vi "PH_PP_CurrentMeas.set i Attr.vi"(0 "i ref in":refnum<vi>, 5 "error in (no error)":errorcluster) -> (14 "i ref out":refnum<vi>, 17 "i Attributes":T1={"Status"={"GUI Ref Hardware Feedback"=refnum, "Tab Control"=refnum}, "PU 1"={"Instance"="N/A", "Status"=0, "Ref Status "=refnum, "Data"=[], "Ref Data"=refnum}, "PU 2"={"Instance"="N/A", "Status"=0, "Ref Status "=refnum, "Data"=[], "Ref Data"=refnum}, "PU 3"={"Instance"="N/A", "Status"=0, "Ref Status "=refnum, "Data"=[], "Ref Data"=refnum}, "PU 4"={"Instance"="N/A", "Status"=0, "Ref Status "=refnum, "Data"=[], "Ref Data"=refnum}, "PU 5"={"Instance"="N/A", "Status"=0, "Ref Status "=refnum, "Data"=[], "Ref Data"=refnum}, "FR"={"Instance"="N/A", "Status"=0, "Ref Status "=refnum, "Data"=[], "Ref Data"=refnum}, "PA - 19mm 1"={"Instance"="N/A", "Status"=0, "Ref Status "=refnum}, "PA - 19mm 2"={"Instance"="N/A", "Status"=0, "Ref Status "=refnum, "no link"=FALSE}, "PA - 45mm"={"Instance"="N/A", "Status"=0, "Ref Status "=refnum, "no link"=FALSE}, "PA Data"={"Data"=[], "Ref"=refnum}, "Sequencer"={"Instance"="N/A", "SM State Ref"=refnum}, "Tasks"=[], "in use"={"MA DP"=FALSE, "FR and PA"=FALSE}, "DAQ Server"="N/A"} {"Tasks"."Status" items=["no info", "off/false/out", "on/true/in", "Failure", "Alarm", "Status 1", "Status 2", "Status 3"]; "PA - 45mm"."Status" items=["no info", "off/false/out", "on/true/in", "Failure", "Alarm", "Status 1", "Status 2", "Status 3"]; "PA - 19mm 2"."Status" items=["no info", "off/false/out", "on/true/in", "Failure", "Alarm", "Status 1", "Status 2", "Status 3"]; "PA - 19mm 1"."Status" items=["no info", "off/false/out", "on/true/in", "Failure", "Alarm", "Status 1", "Status 2", "Status 3"]; "FR"."Status" items=["no info", "off/false/out", "on/true/in", "Failure", "Alarm", "Status 1", "Status 2", "Status 3"]; "PU 5"."Status" items=["no info", "off/false/out", "on/true/in", "Failure", "Alarm", "Status 1", "Status 2", "Status 3"]; "PU 4"."Status" items=["no info", "off/false/out", "on/true/in", "Failure", "Alarm", "Status 1", "Status 2", "Status 3"]; "PU 3"."Status" items=["no info", "off/false/out", "on/true/in", "Failure", "Alarm", "Status 1", "Status 2", "Status 3"]; "PU 2"."Status" items=["no info", "off/false/out", "on/true/in", "Failure", "Alarm", "Status 1", "Status 2", "Status 3"]; "PU 1"."Status" items=["no info", "off/false/out", "on/true/in", "Failure", "Alarm", "Status 1", "Status 2", "Status 3"]}, 19 "error out":errorcluster)   [LabVIEW 2014, in "PH_PP_CurrentMeas.lvlib"]
doc: "Within this VI several Attributes are set the first time."
uses:
  PH_PP_CurrentMeas.lvlib
  PH_PP_CurrentMeas.i attribute.ctl
  PH_Basics/PH_StatusHandler/PH_StatusHandler.Status.ctl
  PH_Basics/PH_StatusHandler/PH_StatusHandler.GUI element.ctl
  PH_PP_CurrentMeas.CommandCluster.ctl
  PH_Basics/PH_StatusHandler/PH_StatusHandler.lvlib
  PH_Basics/PH_Common/PH_Common.lvlib
  CS_Core/CSSystem/CSSystemLib/CSSystemLib.lvlib
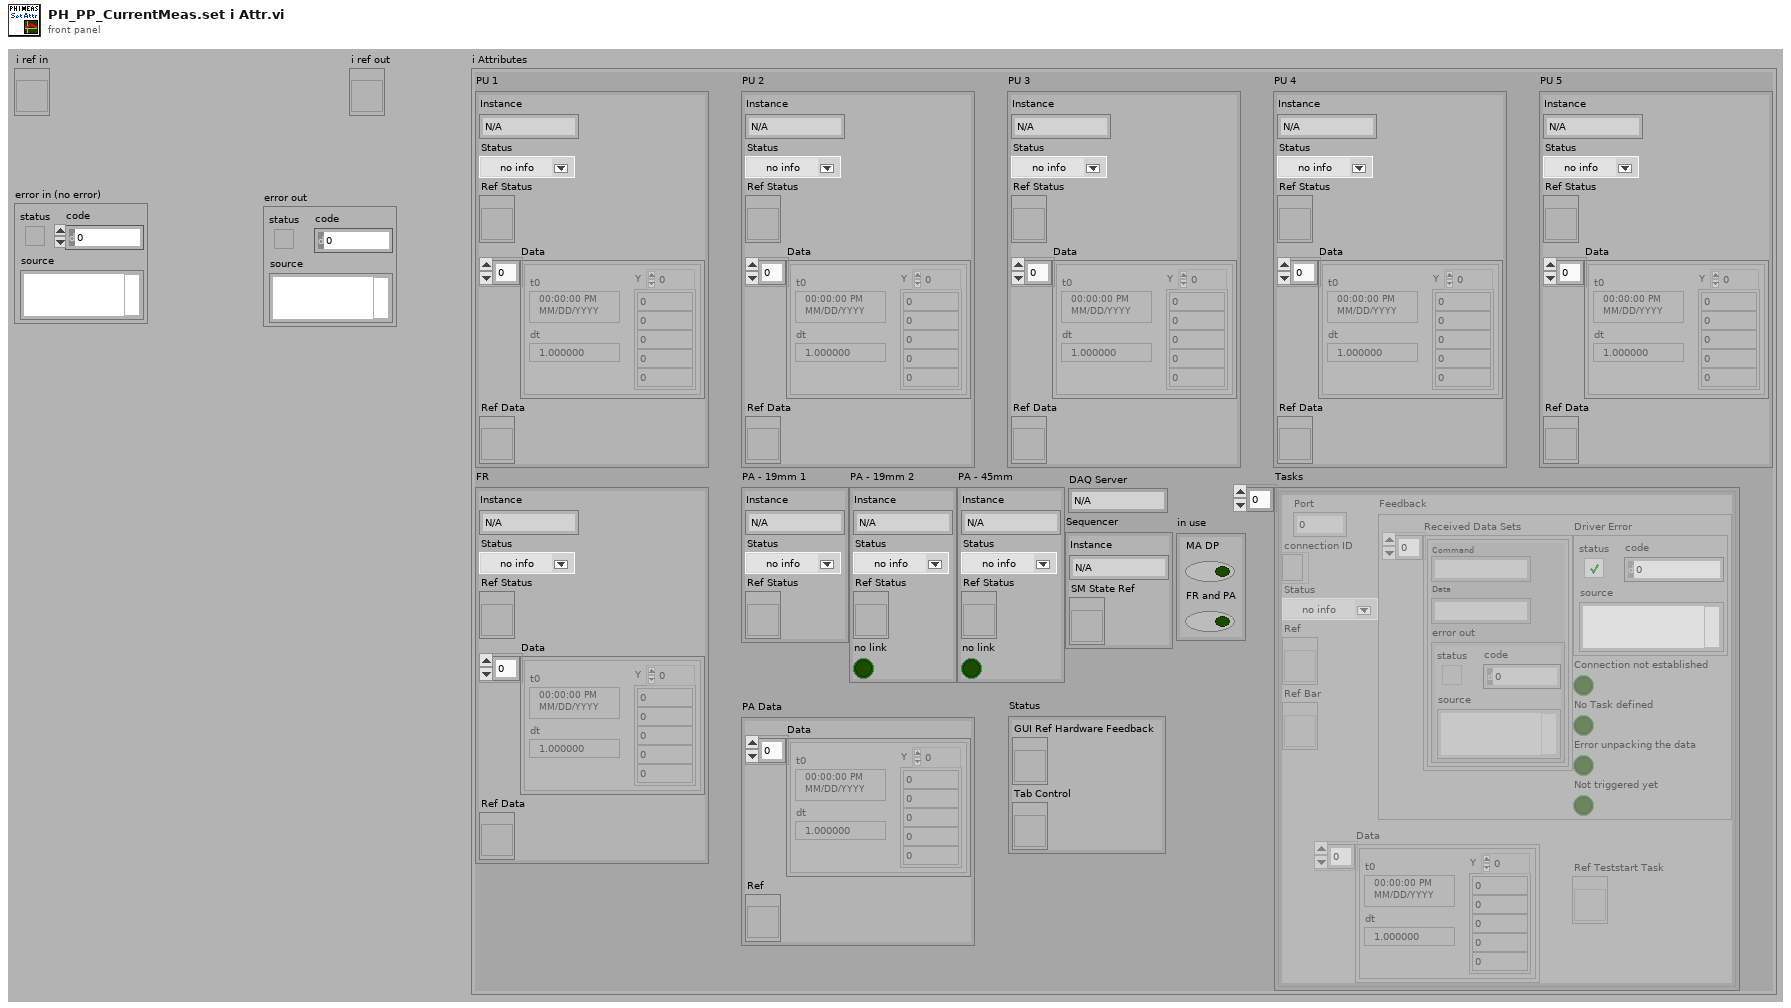
[diagram p1: front panel]
types:
  T1 = typedef "PH_PP_CurrentMeas.lvlib/PH_PP_CurrentMeas.i attribute.ctl" = cluster{"Status":cluster{"GUI Ref Hardware Feedback":refnum<vi>, "Tab Control":refnum<vi>}, "PU 1":cluster{"Instance":string, "Status":T2, "Ref Status ":refnum<vi>, "Data":waveform(dbl)[], "Ref Data":refnum<vi>}, "PU 2":cluster{"Instance":string, "Status":T2, "Ref Status ":refnum<vi>, "Data":waveform(dbl)[], "Ref Data":refnum<vi>}, "PU 3":cluster{"Instance":string, "Status":T2, "Ref Status ":refnum<vi>, "Data":waveform(dbl)[], "Ref Data":refnum<vi>}, "PU 4":cluster{"Instance":string, "Status":T2, "Ref Status ":refnum<vi>, "Data":waveform(dbl)[], "Ref Data":refnum<vi>}, "PU 5":cluster{"Instance":string, "Status":T2, "Ref Status ":refnum<vi>, "Data":waveform(dbl)[], "Ref Data":refnum<vi>}, "FR":cluster{"Instance":string, "Status":T2, "Ref Status ":refnum<vi>, "Data":waveform(dbl)[], "Ref Data":refnum<vi>}, "PA - 19mm 1":cluster{"Instance":string, "Status":T2, "Ref Status ":refnum<vi>}, "PA - 19mm 2":cluster{"Instance":string, "Status":T2, "Ref Status ":refnum<vi>, "no link":bool}, "PA - 45mm":cluster{"Instance":string, "Status":T2, "Ref Status ":refnum<vi>, "no link":bool}, "PA Data":cluster{"Data":waveform(dbl)[], "Ref":refnum<vi>}, "Sequencer":cluster{"Instance":string, "SM State Ref":refnum<vi>}, "Tasks":cluster{"Port":u16, "connection ID":refnum<k5>, "Status":T2, "Ref":refnum<vi>, "Ref Bar":refnum<vi>, "Feedback":cluster{"Received Data Sets":T3[], "Driver Error":errorcluster, "Connection not established":bool, "Error unpacking the data":bool, "No Task defined":bool, "Not triggered yet":bool}, "Data":waveform(dbl)[], "Ref Teststart Task":refnum<vi>}[], "in use":cluster{"MA DP":bool, "FR and PA":bool}, "DAQ Server":string}
  T2 = typedef "PH_StatusHandler.lvlib/PH_StatusHandler.Status.ctl" = i16
  T3 = typedef "PH_PP_CurrentMeas.lvlib/PH_PP_CurrentMeas.CommandCluster.ctl" = cluster{"Command":string, "Data":string, "error out":errorcluster}
  T4 = cluster{"Port":u16, "connection ID":refnum<k5>, "Status":T2, "Ref":refnum<vi>, "Ref Bar":refnum<vi>, "Feedback":cluster{"Received Data Sets":T3[], "Driver Error":errorcluster, "Connection not established":bool, "Error unpacking the data":bool, "No Task defined":bool, "Not triggered yet":bool}, "Data":waveform(dbl)[], "Ref Teststart Task":refnum<vi>}
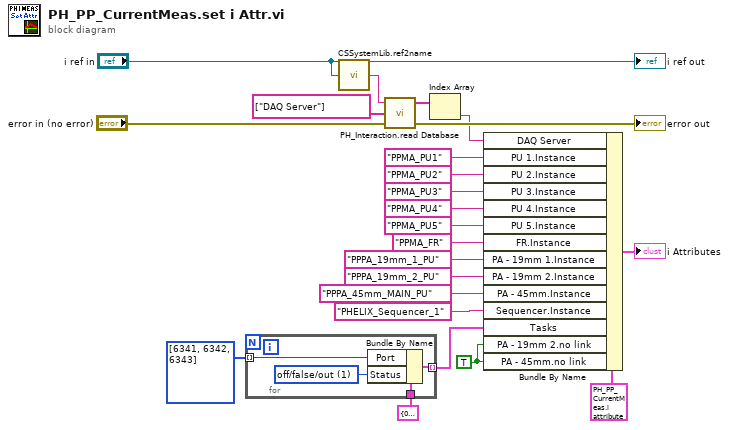
[diagram p0: block diagram]
diagram:
  w3 = TRUE
  n1 = for {
    tunnel: T4 {"Port"=0, "connection ID"=refnum, "Status"=0, "Ref"=refnum, "Ref Bar"=refnum, "Feedback"={"Received Data Sets"=[], "Driver Error"={"status"=FALSE, "code"=0, "source"=""}, "Connection not established"=FALSE, "Error unpacking the data"=FALSE, "No Task defined"=FALSE, "Not triggered yet"=FALSE}, "Data"=[], "Ref Teststart Task"=refnum} ("Task") -> [w27]
    tunnel: [w26] -> w11 mode=indexing
    tunnel: u16[] [6341, 6342, 6343] -> [w25] mode=indexing
    w24 = T2 1 items=["no info", "off/false/out", "on/true/in", "Failure", "Alarm", "Status 1", "Status 2", "Status 3"] ("Status")
    n2 = Bundle By Name(cluster=w27, "Port"=w25, "Status"=w24) -> (w26:T4)
  }
  n3 = call "CSSystemLib.ref2name.vi"("obj refnum"="i ref in") -> ("name"=w4:string)
  n4 = call "PH_Interaction.read Database.vi"("error in (no error)"="error in (no error)", "Strings to search for"=string[] ["DAQ Server"], "DB Entry to read"=w4) -> ("error out"=→"error out":errorcluster, "Values"=w7:string[])  [unwired: 1 in]
  n5 = Index Array(array=w7) -> (element=w6:string)  [unwired: 1 in]
  n6 = Bundle By Name(cluster=T1 {"Status"={"GUI Ref Hardware Feedback"=refnum, "Tab Control"=refnum}, "PU 1"={"Instance"="", "Status"=0, "Ref Status "=refnum, "Data"=[], "Ref Data"=refnum}, "PU 2"={"Instance"="", "Status"=0, "Ref Status "=refnum, "Data"=[], "Ref Data"=refnum}, "PU 3"={"Instance"="", "Status"=0, "Ref Status "=refnum, "Data"=[], "Ref Data"=refnum}, "PU 4"={"Instance"="", "Status"=0, "Ref Status "=refnum, "Data"=[], "Ref Data"=refnum}, "PU 5"={"Instance"="", "Status"=0, "Ref Status "=refnum, "Data"=[], "Ref Data"=refnum}, "FR"={"Instance"="", "Status"=0, "Ref Status "=refnum, "Data"=[], "Ref Data"=refnum}, "PA - 19mm 1"={"Instance"="", "Status"=0, "Ref Status "=refnum}, "PA - 19mm 2"={"Instance"="", "Status"=0, "Ref Status "=refnum, "no link"=FALSE}, "PA - 45mm"={"Instance"="", "Status"=0, "Ref Status "=refnum, "no link"=FALSE}, "PA Data"={"Data"=[], "Ref"=refnum}, "Sequencer"={"Instance"="", "SM State Ref"=refnum}, "Tasks"=[], "in use"={"MA DP"=FALSE, "FR and PA"=FALSE}, "DAQ Server"=""} ("i attribute"), "DAQ Server"=w6, "PU 1.Instance"="PPMA_PU1", "PU 2.Instance"="PPMA_PU2", "PU 3.Instance"="PPMA_PU3", "PU 4.Instance"="PPMA_PU4", "PU 5.Instance"="PPMA_PU5", "FR.Instance"="PPMA_FR", "PA - 19mm 1.Instance"="PPPA_19mm_1_PU", "PA - 19mm 2.Instance"="PPPA_19mm_2_PU", "PA - 45mm.Instance"="PPPA_45mm_MAIN_PU", "Sequencer.Instance"="PHELIX_Sequencer_1", "Tasks"=w11, "PA - 19mm 2.no link"=w3, "PA - 45mm.no link"=w3) -> (→"i Attributes":T1)
  "i ref out" <- "i ref in"
